vi "Write Connection Event.vi"(8 "error in (no error)":errorcluster, 10 "Connection Event":T1, 11 "WebSocket Connection Handler Msg in":refnum<class "WebSocket Connection Handler Msg.lvclass">) -> (0 "error out":errorcluster, 3 "WebSocket Connection Handler Msg out":refnum<class "WebSocket Connection Handler Msg.lvclass">)   [LabVIEW 2016, in "WebSocket Actors.lvlib" / "WebSocket Connection Handler Msg.lvclass"]
uses:
  WebSocket Connection Handler Msg.lvclass
  Connection Event.ctl
  WebSocket Connection Handler Msg.lvclass/WebSocket Connection Handler Msg.ctl
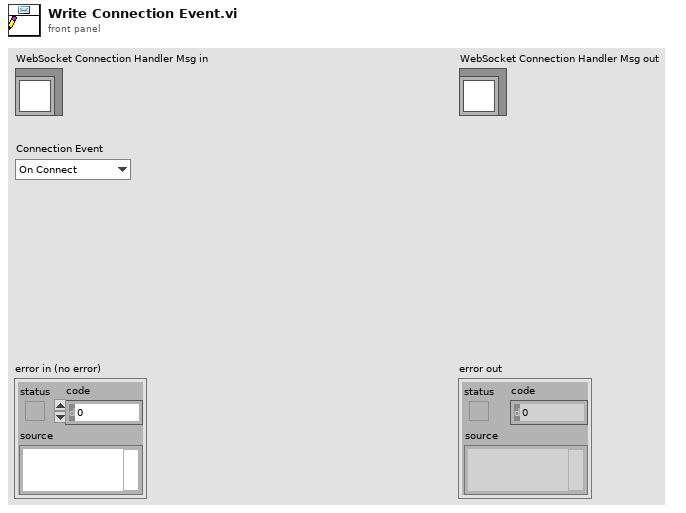
[diagram p1: front panel]
types:
  T1 = typedef "WebSocket Actors.lvlib/WebSocket Connection Handler Msg.lvclass/Connection Event.ctl" = enum16{"On Connect", "On Message", "On Close"}
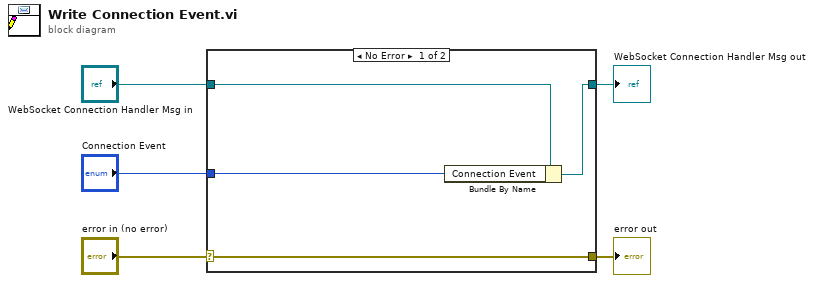
[diagram p0: block diagram]
diagram:
  n1 = case shown="No Error" "error in (no error)" {
    selector: "error in (no error)" -> [w9 w10]
    tunnel: [w9 w10] -> w4
    tunnel: [w7 w11] -> w2
    tunnel: "WebSocket Connection Handler Msg in" -> [w8 w11]
    tunnel: "Connection Event" -> [w6 _]
    frame No Error {
      n2 = Bundle By Name(cluster=w8, "Connection Event"=w6) -> (w7:refnum<class "WebSocket Connection Handler Msg.lvclass">)
    }
    frame Error {
    }
  }
  "error out" <- w4
  "WebSocket Connection Handler Msg out" <- w2
